vi "Get Time Date String.vi"() -> (0 "String":string)   [LabVIEW 2012, in "Strings Lib.lvlib"]
uses:
  Strings Lib.lvlib
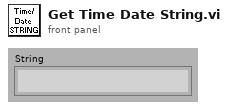
[diagram p1: front panel]
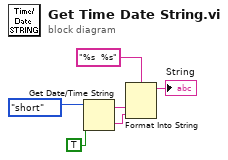
[diagram p0: block diagram]
diagram:
  n1 = Get Date/Time String(date format (0)=enum16{"short", "long", "abbreviated"}."short", want seconds? (F)=TRUE) -> (date string=w3:string, time string=w4:string)  [unwired: 1 out]
  n2 = Format Into String(format string="%s  %s", w3, w4) -> (resulting string=→"String":string)  [unwired: 2 in, 1 out]
